vi "FullSpectrum.vi"(9 "Rotating Direction":u16(ring) items=["CCW", "CW"], 10 "Channel 2":waveform(sgl), 11 "Channel 1":waveform(sgl)) -> (3 "Full Spectrum (EU rms)":cluster{"f0":dbl, "df":dbl, "magnitude":dbl[]}, 4 "Crude Orbit (assumes exactly orthogonal)":T1, 5 "Ch2 Spectrum (EU rms)":cluster{"f0":dbl, "df":dbl, "magnitude":dbl[]}, 7 "Ch 1 Spectrum (EU rms)":cluster{"f0":dbl, "df":dbl, "magnitude":dbl[]})   [LabVIEW 2017, in "VibrationAnalysisFunctions.lvlib"]
uses:
  <vilib>/addons/InsightCM/Utilities/Analysis/Vibration/VibrationAnalysisFunctions.lvlib
  <vilib>/addons/_NISVFA/_Shared subVIs/Controls/svc_Window [Dual FFT].ctl
  <vilib>/addons/_NISVFA/_Baseband FFT/SVPO Power Spectrum (1 Ch DBL Array).vi
  <vilib>/addons/_NISVFA/_Baseband FFT/subVIs/svfa_Convert to One-Sided Power Spectrum.vi
  <vilib>/Analysis/2dsp.llb/Power Spectrum.vi
  <vilib>/Analysis/2dsp.llb/Power Spectrum (DBL).vi
  <vilib>/addons/_NISVFA/_Shared subVIs/Windowing/svfa_Scaled Time Domain Window (Array).vi
  <vilib>/Analysis/4window.llb/Force Window.vi
  <vilib>/Analysis/4window.llb/Force Window (DBL).vi
  <vilib>/Analysis/4window.llb/Exponential Window.vi
  <vilib>/Analysis/4window.llb/Exponential Window (DBL).vi
  <vilib>/addons/_NISVFA/_Spectrum Processing/subVIs/svfa_Spectrum Info Window to windowTd Type Def.vi
  <vilib>/Analysis/0measdsp.llb/Scaled Time Domain Window.vi
  <vilib>/Analysis/0measdsp.llb/Scaled Time Domain Window (DBL).vi
  <vilib>/Utility/error.llb/Error Cluster From Error Code.vi
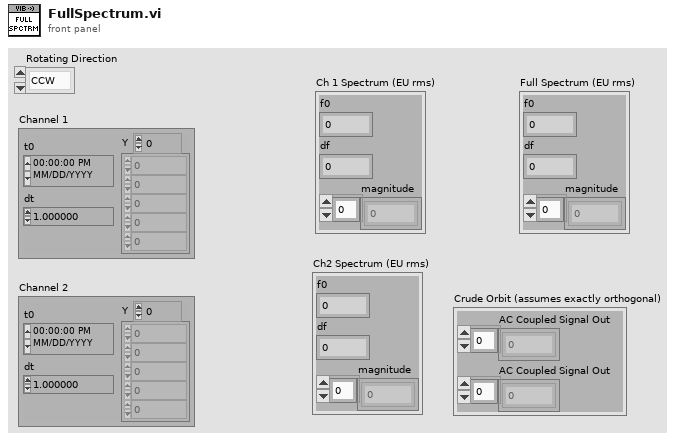
[diagram p1: front panel]
types:
  T1 = cluster{"AC Coupled Signal Out":sgl[], "AC Coupled Signal Out":sgl[]}
  T2 = typedef "svc_Window [Dual FFT].ctl" = u32
  T3 = cluster{"dB On (T)":bool, "unwrap phase (F)":bool, "convert to degree (T)":bool}
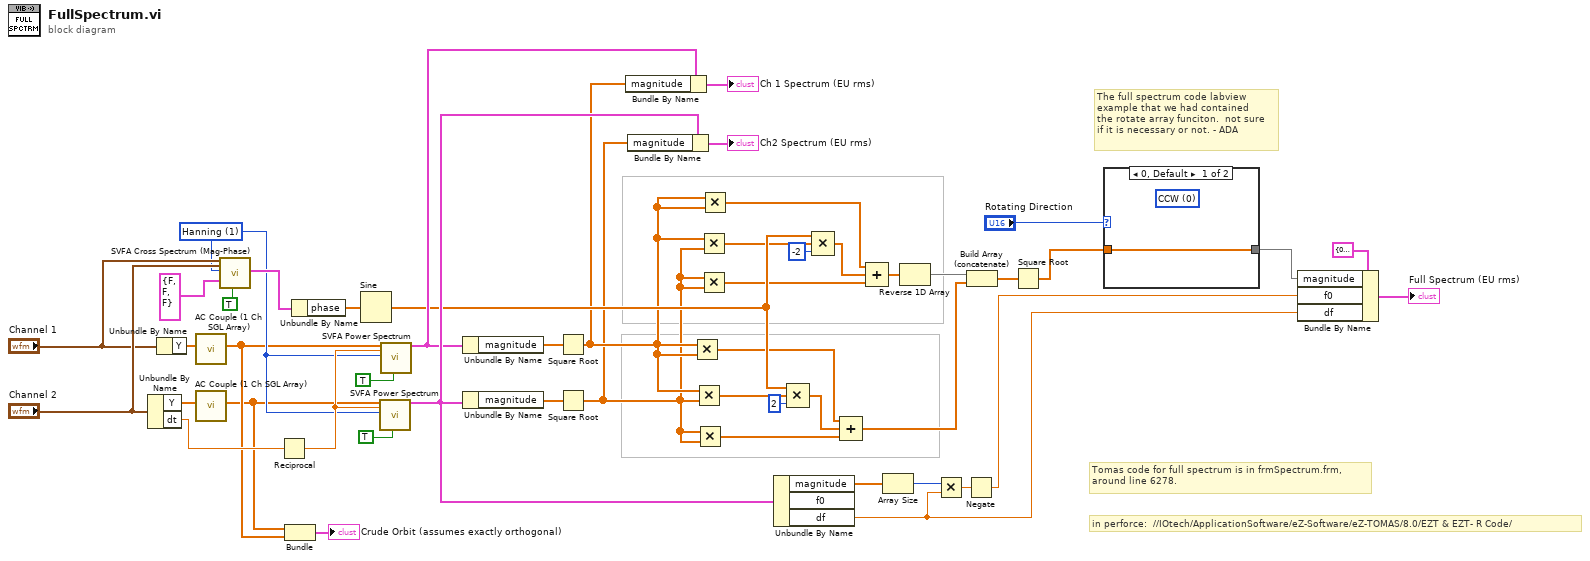
[diagram p0: block diagram]
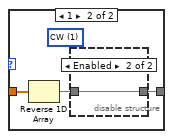
[diagram p2: hidden frame]
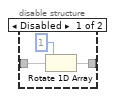
[diagram p3: hidden frame]
diagram:
  w12 = T2 1 items=["None"=0, "Hanning"=1, "Hamming"=2, "Blackman-Harris"=3, "Exact Blackman"=4, "Blackman"=5, "Flat Top"=6, "4 Term B-Harris "=7, "7 Term B-Harris"=8, "Low Sidelobe"=9, "Force - Exponential"=10, "Blackman Nuttall"=11, "Triangle"=30, "Bartlett-Hanning"=31, "Bohman"=32, "Parzen"=33, "Welch"=34, "Kaiser"=60, "Dolph-Chebyshev"=61, "Gaussian"=62] ("window")
  # "in perforce:  //IOtech/ApplicationSoftware/eZ-Software/eZ-TOMAS/8.0/EZT & EZT- R Code/"
  # "Tomas code for full spectrum is in frmSpectrum.frm,\naround line 6278."
  # "The full spectrum code labview\nexample that we had contained\nthe rotate array funciton.  not sure\nif it is necessary or not. - ADA"
  n1 = Unbundle By Name("Channel 2") -> ("Y"=w2:sgl[], "dt"=w13:dbl)
  n2 = Unbundle By Name("Channel 1") -> ("Y"=w4:sgl[])
  n3 = call <vilib>:"AC Couple (1 Ch SGL Array).vi"("Signal"=w4) -> ("AC Coupled"=w3:sgl[])  [unwired: 8 in, 2 out]
  n4 = call <vilib>:"AC Couple (1 Ch SGL Array).vi"("Signal"=w2) -> ("AC Coupled"=w1:sgl[])  [unwired: 8 in, 2 out]
  n5 = call <vilib>:"SVFA Cross Spectrum (Mag-Phase).vi"("scaled signal X [EUx]"="Channel 1", "scaled signal Y [EUy]"="Channel 2", "window"=w12, "view"=T3 {"dB On (T)"=FALSE, "unwrap phase (F)"=FALSE, "convert to degree (T)"=FALSE}, "restart averaging (F)"=TRUE) -> ("phase [degrees]"=w32:cluster{"f0":dbl, "df":dbl, "phase":dbl[]})  [unwired: 7 in, 7 out]
  n6 = Reciprocal(x=w13) -> (1/x=w35:dbl)
  n7 = Bundle("AC Coupled"=w1, "AC Coupled"=w3) -> (→"Crude Orbit (assumes exactly orthogonal)":cluster{"AC Coupled":sgl[], "AC Coupled":sgl[]})  [unwired: 1 in]
  n8 = Unbundle By Name(w32) -> ("phase"=w34:dbl[])
  n9 = Sine(x=w34) -> (sin(x)=w28:dbl[])
  n10 = call-poly <vilib>:"SVFA Power Spectrum.vi"("scaled signal [EU]"=w1, "sampling rate [Hz]"=w35, "window"=w12, "restart averaging? (F)"=TRUE) -> ("power spectrum [EU^2 rms]"=w47:cluster{"f0":dbl, "df":dbl, "magnitude":dbl[]})  [unwired: 13 in, 2 out]
  n11 = call-poly <vilib>:"SVFA Power Spectrum.vi"("scaled signal [EU]"=w3, "sampling rate [Hz]"=w35, "window"=w12, "restart averaging? (F)"=TRUE) -> ("power spectrum [EU^2 rms]"=w44:cluster{"f0":dbl, "df":dbl, "magnitude":dbl[]})  [unwired: 13 in, 2 out]
  n12 = Unbundle By Name(w44) -> ("magnitude"=w37:dbl[])
  n13 = Unbundle By Name(w47) -> ("magnitude"=w45:dbl[])
  n14 = Square Root(x=w37) -> (sqrt(x)=w9:dbl[])
  n15 = Square Root(x=w45) -> (sqrt(x)=w8:dbl[])
  n16 = Bundle By Name(cluster=w44, "magnitude"=w9) -> (→"Ch 1 Spectrum (EU rms)":cluster{"f0":dbl, "df":dbl, "magnitude":dbl[]})
  n17 = Bundle By Name(cluster=w47, "magnitude"=w8) -> (→"Ch2 Spectrum (EU rms)":cluster{"f0":dbl, "df":dbl, "magnitude":dbl[]})
  n18 = Multiply(x=w9, y=w9) -> (x*y=w19:dbl[])
  n19 = Multiply(x=w9, y=w8) -> (x*y=w21:dbl[])
  n20 = Multiply(x=w8, y=w8) -> (x*y=w20:dbl[])
  n21 = Multiply(x=w9, y=w8) -> (x*y=w23:dbl[])
  n22 = Multiply(x=w8, y=w8) -> (x*y=w24:dbl[])
  n23 = Multiply(x=w9, y=w9) -> (x*y=w25:dbl[])
  n24 = Unbundle By Name(w47) -> ("magnitude"=w46:dbl[], "df"=w10:dbl)  [unwired: 1 out]
  n25 = Compound Arithmetic op=MULTIPLY(w28, w21, 2 ("index (page)")) -> (w18:dbl[])
  n26 = Compound Arithmetic op=MULTIPLY(w28, w23, -2 ("index (page)")) -> (w26:dbl[])
  n27 = Compound Arithmetic op=ADD(w19, w18, w20) -> (w43:dbl[])
  n28 = Compound Arithmetic op=ADD(w25, w26, w24) -> (w42:dbl[])
  n29 = Array Size(array=w46) -> (size(s)=w48:i32)
  n30 = Reverse 1D Array(array=w42) -> (reversed array=w29:dbl[])
  n31 = Multiply(x=w48, y=w10) -> (x*y=w49:dbl)
  n32 = Negate(x=w49) -> (-x=w11:dbl)
  n33 = Build Array (concatenate)(w29, w43) -> (w39:dbl[])
  n34 = Square Root(x=w39) -> (sqrt(x)=w6:dbl[])
  n35 = case shown="0, Default" "Rotating Direction" {
    tunnel: [w50 w51] -> w7
    tunnel: w6 -> [w50 w52]
    frame 0, Default {
      (unwired) u16 0 items=["CCW", "CW"] ("Rotating Direction 2")
    }
    frame 1 {
      (unwired) u16 1 items=["CCW", "CW"] ("Rotating Direction 2")
      n36 = Reverse 1D Array(array=w52) -> (reversed array=w53:dbl[])
      n37 = disable-structure shown="Enabled" {
        disable-tunnel: w53 -> [w56 w57]
        disable-tunnel: [w54 w57] -> w51
        frame Disabled {
          n38 = Rotate 1D Array(1:w56, 2:1 ("n")) -> (0:w54:dbl[])
        }
        frame Enabled {
        }
      }
    }
  }
  n39 = Bundle By Name(cluster=cluster{"f0":dbl, "df":dbl, "magnitude":dbl[]} {"f0"=0.0, "df"=0.0, "magnitude"=[]} ("magnitude [dB EUx EUy]"), "magnitude"=w7, "f0"=w11, "df"=w10) -> (→"Full Spectrum (EU rms)":cluster{"f0":dbl, "df":dbl, "magnitude":dbl[]})
